vi "Configure Trigger Output.vi"(7 "Output Trigger Source (0: CH1)":i32(ring) items=["CH1", "CH2"], 8 "error in (no error)":errorcluster, 9 "Trigger Slope (0: Positive)":i32(ring) items=["Positive", "Negative"], 10 "Enable Trigger Output (T: Enable)":bool=TRUE, 11 "VISA resource name":refnum<visa-resource-name>) -> (0 "error out":errorcluster, 3 "VISA resource name out":refnum<visa-resource-name>)   [LabVIEW 2020, in "AWG.lvlib" / "Agilent 3352X Series.lvlib"]
doc: "Enables and configures output trigger.\nIncluding source setting and slope setting."
uses:
  Agilent 3352X Series.lvlib
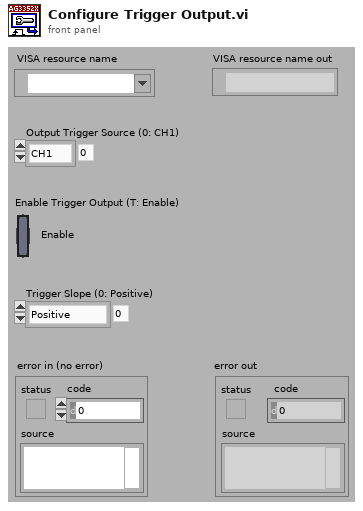
[diagram p1: front panel]
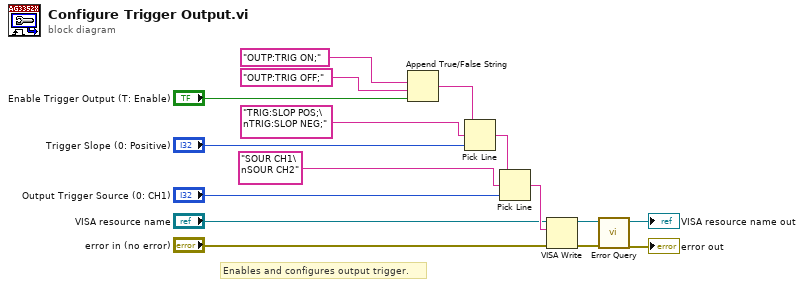
[diagram p0: block diagram]
diagram:
  # "Enables and configures output trigger."
  n1 = Append True/False String(1:"Enable Trigger Output (T: Enable)", 2:"OUTP:TRIG OFF;", 3:"OUTP:TRIG ON;") -> (0:w1:string)  [unwired: 1 out]
  n2 = Pick Line(string ("")=w1, multi-line string="TRIG:SLOP POS;\nTRIG:SLOP NEG;", line index="Trigger Slope (0: Positive)") -> (output string=w12:string)
  n3 = Pick Line(string ("")=w12, multi-line string="SOUR CH1\nSOUR CH2", line index="Output Trigger Source (0: CH1)") -> (output string=w11:string)
  n4 = VISA Write(VISA resource name="VISA resource name", write buffer=w11, error in (no error)="error in (no error)") -> (VISA resource name out=w8:refnum<visa-resource-name>, error out=w7:errorcluster)  [unwired: 1 out]
  n5 = call "Error Query.vi"("error in (no error)"=w7, "VISA resource name"=w8) -> ("error out"=→"error out":errorcluster, "VISA resource name out"=→"VISA resource name out":refnum<visa-resource-name>)  [unwired: 8 out]
